vi "HEWH Agilent Data Output.vi"(8 "error in (no error)":errorcluster, 10 "Output Array in":dbl[](array[numeric])) -> (0 "error out":errorcluster, 3 "Agilent Data":T1)   [LabVIEW 2023]
uses:
  Type Definitions/HEWH Agilent Data.ctl
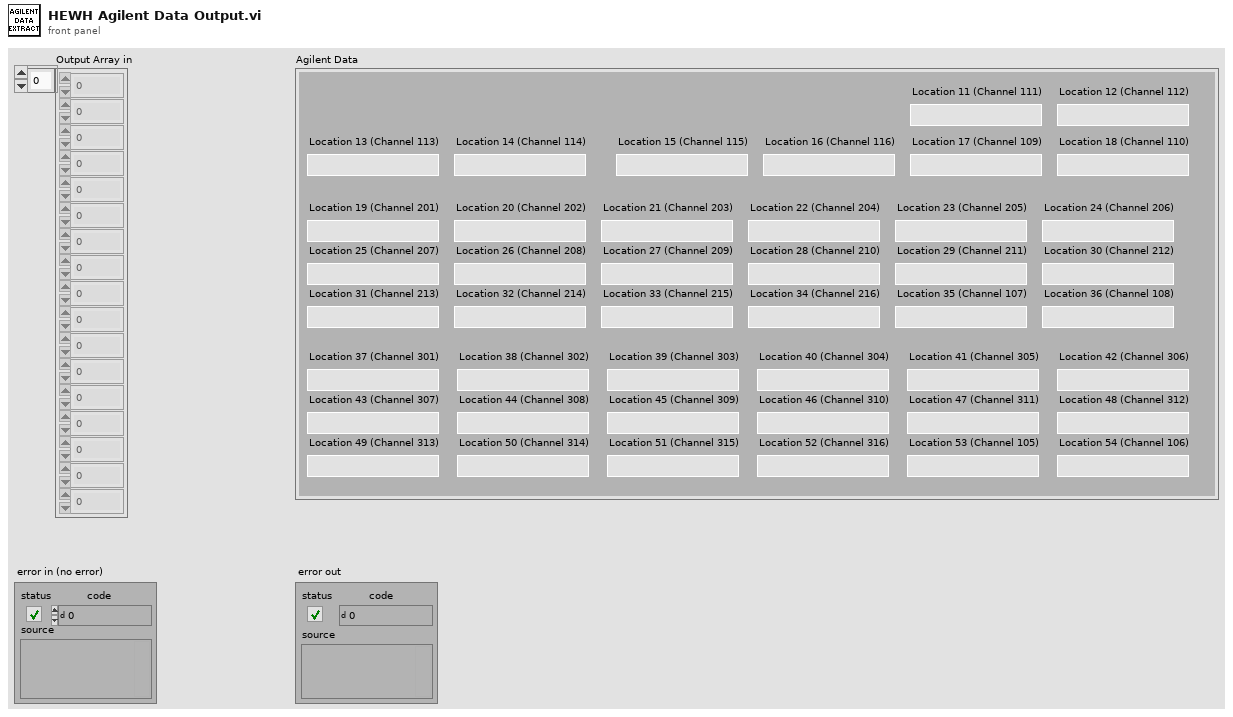
[diagram p1: front panel]
types:
  T1 = typedef "HEWH Agilent Data.ctl" = cluster{"Location 11 (Channel 111)":dbl, "Location 12 (Channel 112)":dbl, "Location 13 (Channel 113)":dbl, "Location 14 (Channel 114)":dbl, "Location 15 (Channel 115)":dbl, "Location 16 (Channel 116)":dbl, "Location 17 (Channel 109)":dbl, "Location 18 (Channel 110)":dbl, "Location 19 (Channel 201)":dbl, "Location 20 (Channel 202)":dbl, "Location 21 (Channel 203)":dbl, "Location 22 (Channel 204)":dbl, "Location 23 (Channel 205)":dbl, "Location 24 (Channel 206)":dbl, "Location 25 (Channel 207)":dbl, "Location 26 (Channel 208)":dbl, "Location 27 (Channel 209)":dbl, "Location 28 (Channel 210)":dbl, "Location 29 (Channel 211)":dbl, "Location 30 (Channel 212)":dbl, "Location 31 (Channel 213)":dbl, "Location 32 (Channel 214)":dbl, "Location 33 (Channel 215)":dbl, "Location 34 (Channel 216)":dbl, "Location 35 (Channel 107)":dbl, "Location 36 (Channel 108)":dbl, "Location 37 (Channel 301)":dbl, "Location 38 (Channel 302)":dbl, "Location 39 (Channel 303)":dbl, "Location 40 (Channel 304)":dbl, "Location 41 (Channel 305)":dbl, "Location 42 (Channel 306)":dbl, "Location 43 (Channel 307)":dbl, "Location 44 (Channel 308)":dbl, "Location 45 (Channel 309)":dbl, "Location 46 (Channel 310)":dbl, "Location 47 (Channel 311)":dbl, "Location 48 (Channel 312)":dbl, "Location 49 (Channel 313)":dbl, "Location 50 (Channel 314)":dbl, "Location 51 (Channel 315)":dbl, "Location 52 (Channel 316)":dbl, "Location 53 (Channel 105)":dbl, "Location 54 (Channel 106)":dbl}
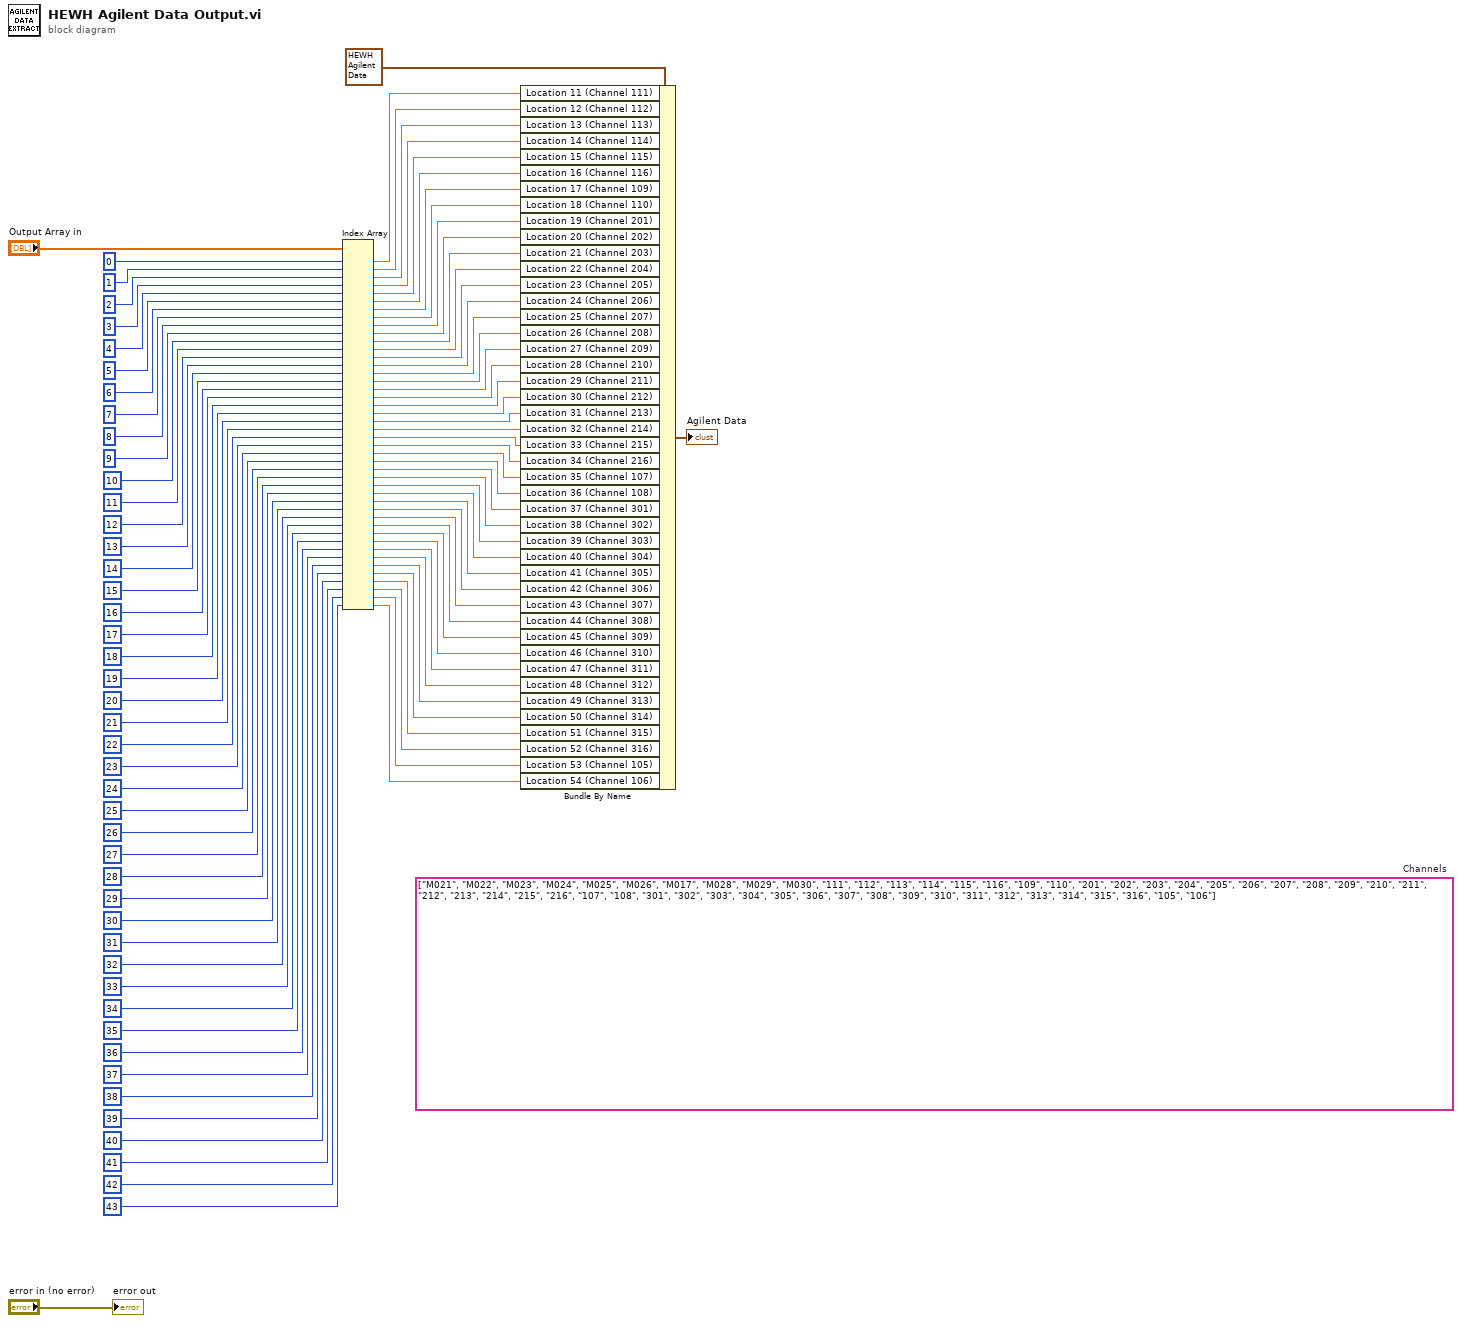
[diagram p0: block diagram]
diagram:
  (unwired) string[][] [["M021", "M022", "M023", "M024", "M025", "M026"], ["M017", "M028", "M029", "M030", "111", "112"], ["113", "114", "115", "116", "109", "110"], ["201", "202", "203", "204", "205", "206"], ["207", "208", "209", "210", "211", "212"], ["213", "214", "215", "216", "107", "108"], ["301", "302", "303", "304", "305", "306"], ["307", "308", "309", "310", "311", "312"], ["313", "314", "315", "316", "105", "106"]]  # Channels
  n1 = Index Array(array="Output Array in", index #1=0 ("index"), index #2=1 ("index"), index #3=2 ("index"), index #4=3 ("index"), index #5=4 ("index"), index #6=5 ("index"), index #7=6 ("index"), index #8=7 ("index"), index #9=8 ("index"), index #10=9 ("index"), index #11=10 ("index"), index #12=11 ("index"), index #13=12 ("index"), index #14=13 ("index"), index #15=14 ("index"), index #16=15 ("index"), index #17=16 ("index"), index #18=17 ("index"), index #19=18 ("index"), index #20=19 ("index"), index #21=20 ("index"), index #22=21 ("index"), index #23=22 ("index"), index #24=23 ("index"), index #25=24 ("index"), index #26=25 ("index"), index #27=26 ("index"), index #28=27 ("index"), index #29=28 ("index"), index #30=29 ("index"), index #31=30 ("index"), index #32=31 ("index"), index #33=32 ("index"), index #34=33 ("index"), index #35=34 ("index"), index #36=35 ("index"), index #37=36 ("index"), index #38=37 ("index"), index #39=38 ("index"), index #40=39 ("index"), index #41=40 ("index"), index #42=41 ("index"), index #43=42 ("index"), index #44=43 ("index")) -> (element #1=w88:dbl, element #2=w87:dbl, element #3=w86:dbl, element #4=w85:dbl, element #5=w84:dbl, element #6=w83:dbl, element #7=w82:dbl, element #8=w81:dbl, element #9=w80:dbl, element #10=w79:dbl, element #11=w78:dbl, element #12=w77:dbl, element #13=w76:dbl, element #14=w75:dbl, element #15=w74:dbl, element #16=w73:dbl, element #17=w72:dbl, element #18=w71:dbl, element #19=w70:dbl, element #20=w69:dbl, element #21=w68:dbl, element #22=w67:dbl, element #23=w66:dbl, element #24=w65:dbl, element #25=w64:dbl, element #26=w63:dbl, element #27=w62:dbl, element #28=w61:dbl, element #29=w60:dbl, element #30=w59:dbl, element #31=w58:dbl, element #32=w57:dbl, element #33=w56:dbl, element #34=w55:dbl, element #35=w54:dbl, element #36=w53:dbl, element #37=w52:dbl, element #38=w51:dbl, element #39=w50:dbl, element #40=w49:dbl, element #41=w48:dbl, element #42=w47:dbl, element #43=w46:dbl, element #44=w45:dbl)
  n2 = Bundle By Name(cluster=T1 {"Location 11 (Channel 111)"=0.0, "Location 12 (Channel 112)"=0.0, "Location 13 (Channel 113)"=0.0, "Location 14 (Channel 114)"=0.0, "Location 15 (Channel 115)"=0.0, "Location 16 (Channel 116)"=0.0, "Location 17 (Channel 109)"=0.0, "Location 18 (Channel 110)"=0.0, "Location 19 (Channel 201)"=0.0, "Location 20 (Channel 202)"=0.0, "Location 21 (Channel 203)"=0.0, "Location 22 (Channel 204)"=0.0, "Location 23 (Channel 205)"=0.0, "Location 24 (Channel 206)"=0.0, "Location 25 (Channel 207)"=0.0, "Location 26 (Channel 208)"=0.0, "Location 27 (Channel 209)"=0.0, "Location 28 (Channel 210)"=0.0, "Location 29 (Channel 211)"=0.0, "Location 30 (Channel 212)"=0.0, "Location 31 (Channel 213)"=0.0, "Location 32 (Channel 214)"=0.0, "Location 33 (Channel 215)"=0.0, "Location 34 (Channel 216)"=0.0, "Location 35 (Channel 107)"=0.0, "Location 36 (Channel 108)"=0.0, "Location 37 (Channel 301)"=0.0, "Location 38 (Channel 302)"=0.0, "Location 39 (Channel 303)"=0.0, "Location 40 (Channel 304)"=0.0, "Location 41 (Channel 305)"=0.0, "Location 42 (Channel 306)"=0.0, "Location 43 (Channel 307)"=0.0, "Location 44 (Channel 308)"=0.0, "Location 45 (Channel 309)"=0.0, "Location 46 (Channel 310)"=0.0, "Location 47 (Channel 311)"=0.0, "Location 48 (Channel 312)"=0.0, "Location 49 (Channel 313)"=0.0, "Location 50 (Channel 314)"=0.0, "Location 51 (Channel 315)"=0.0, "Location 52 (Channel 316)"=0.0, "Location 53 (Channel 105)"=0.0, "Location 54 (Channel 106)"=0.0} ("Agilent Data"), "Location 11 (Channel 111)"=w88, "Location 12 (Channel 112)"=w87, "Location 13 (Channel 113)"=w86, "Location 14 (Channel 114)"=w85, "Location 15 (Channel 115)"=w84, "Location 16 (Channel 116)"=w83, "Location 17 (Channel 109)"=w82, "Location 18 (Channel 110)"=w81, "Location 19 (Channel 201)"=w80, "Location 20 (Channel 202)"=w79, "Location 21 (Channel 203)"=w78, "Location 22 (Channel 204)"=w77, "Location 23 (Channel 205)"=w76, "Location 24 (Channel 206)"=w75, "Location 25 (Channel 207)"=w74, "Location 26 (Channel 208)"=w73, "Location 27 (Channel 209)"=w72, "Location 28 (Channel 210)"=w71, "Location 29 (Channel 211)"=w70, "Location 30 (Channel 212)"=w69, "Location 31 (Channel 213)"=w68, "Location 32 (Channel 214)"=w67, "Location 33 (Channel 215)"=w66, "Location 34 (Channel 216)"=w65, "Location 35 (Channel 107)"=w64, "Location 36 (Channel 108)"=w63, "Location 37 (Channel 301)"=w62, "Location 38 (Channel 302)"=w61, "Location 39 (Channel 303)"=w60, "Location 40 (Channel 304)"=w59, "Location 41 (Channel 305)"=w58, "Location 42 (Channel 306)"=w57, "Location 43 (Channel 307)"=w56, "Location 44 (Channel 308)"=w55, "Location 45 (Channel 309)"=w54, "Location 46 (Channel 310)"=w53, "Location 47 (Channel 311)"=w52, "Location 48 (Channel 312)"=w51, "Location 49 (Channel 313)"=w50, "Location 50 (Channel 314)"=w49, "Location 51 (Channel 315)"=w48, "Location 52 (Channel 316)"=w47, "Location 53 (Channel 105)"=w46, "Location 54 (Channel 106)"=w45) -> (→"Agilent Data":T1)
  "error out" <- "error in (no error)"
